vi "OP60_Data.vi"(2 "subarray":string[](array[string])) -> (0 "OP30_VERIFY_STN":T1)   [LabVIEW 2020]
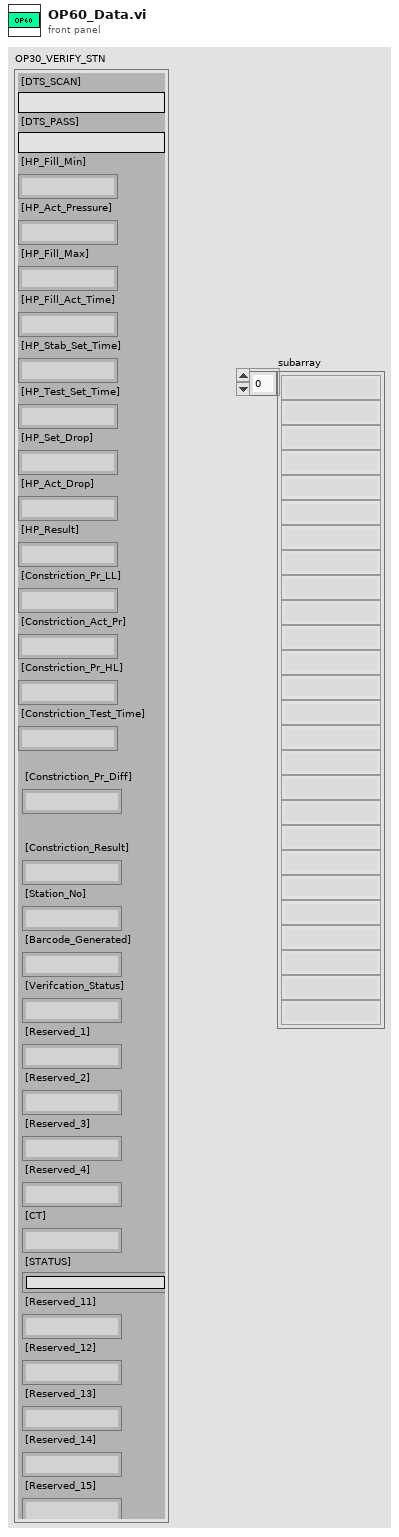
[diagram p1: front panel]
types:
  T1 = cluster{"[DTS_SCAN]":string, "[DTS_PASS]":string, "[HP_Fill_Min]":string, "[HP_Act_Pressure]":string, "[HP_Fill_Max]":string, "[HP_Fill_Act_Time]":string, "[HP_Stab_Set_Time]":string, "[HP_Test_Set_Time]":string, "[HP_Set_Drop]":string, "[HP_Act_Drop]":string, "[HP_Result]":string, "[Constriction_Pr_LL]":string, "[Constriction_Act_Pr]":string, "[Constriction_Pr_HL]":string, "[Constriction_Test_Time]":string, "[Constriction_Pr_Diff]":string, "[Constriction_Result]":string, "[Station_No]":string, "[Barcode_Generated]":string, "[Verifcation_Status]":string, "[Reserved_1]":string, "[Reserved_2]":string, "[Reserved_3]":string, "[Reserved_4]":string, "[CT]":string, "[STATUS]":string, "[Reserved_11]":string, "[Reserved_12]":string, "[Reserved_13]":string, "[Reserved_14]":string, "[Reserved_15]":string}
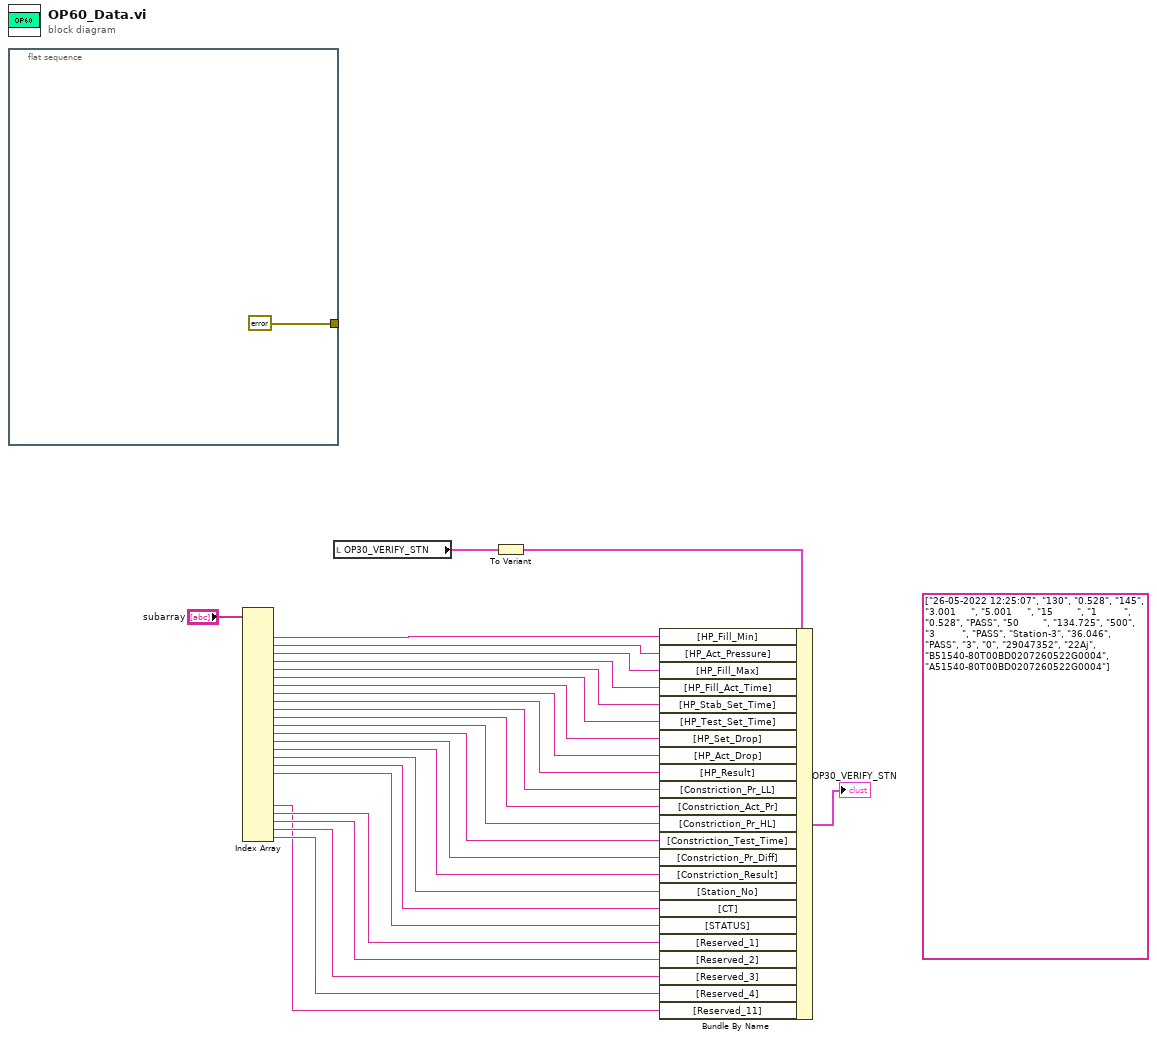
[diagram p0: block diagram]
diagram:
  (unwired) string[] ["26-05-2022 12:25:07", "130", "0.528", "145", "3.001     ", "5.001     ", "15        ", "1         ", "0.528", "PASS", "50        ", "134.725", "500", "3         ", "PASS", "Station-3", "36.046", "PASS", "3", "0", "29047352", "22Aj", "B51540-80T00BD0207260522G0004", "A51540-80T00BD0207260522G0004"] ("subarray")
  n1 = flat-sequence {
    tunnel: [errorcluster {"status"=FALSE, "code"=0, "source"=""} ("error in (no error)")] -> _
    frame #0 {
    }
  }
  n2 = Index Array(array="subarray") -> (element #2=w24:string, element #3=w23:string, element #4=w22:string, element #5=w21:string, element #6=w20:string, element #7=w18:string, element #8=w17:string, element #9=w16:string, element #10=w15:string, element #11=w14:string, element #12=w13:string, element #13=w12:string, element #14=w11:string, element #15=w9:string, element #16=w8:string, element #17=w7:string, element #18=w6:string, element #19=w10:string, element #23=w1:string, element #24=w2:string, element #25=w3:string, element #26=w4:string, element #27=w5:string)  [unwired: 27 in, 4 out]
  n3 = local read "OP30_VERIFY_STN"() -> (w25:T1)
  n4 = To Variant(anything=w25) -> ()  [unwired: 1 out]
  n5 = Bundle By Name(cluster=w25, "[HP_Fill_Min]"=w24, "[HP_Act_Pressure]"=w23, "[HP_Fill_Max]"=w22, "[HP_Fill_Act_Time]"=w21, "[HP_Stab_Set_Time]"=w20, "[HP_Test_Set_Time]"=w18, "[HP_Set_Drop]"=w17, "[HP_Act_Drop]"=w16, "[HP_Result]"=w15, "[Constriction_Pr_LL]"=w14, "[Constriction_Act_Pr]"=w13, "[Constriction_Pr_HL]"=w12, "[Constriction_Test_Time]"=w11, "[Constriction_Pr_Diff]"=w9, "[Constriction_Result]"=w8, "[Station_No]"=w7, "[CT]"=w6, "[STATUS]"=w10, "[Reserved_1]"=w2, "[Reserved_2]"=w3, "[Reserved_3]"=w4, "[Reserved_4]"=w5, "[Reserved_11]"=w1) -> (→"OP30_VERIFY_STN":T1)
